vi "Teleop.vi"(10 "Match Info":T2={"Autonomous Elapsed Seconds"=0.0, "TeleOp Elapsed Seconds"=0.0, "Disabled Elapsed Seconds"=0.0, "Visited Autonomous"=FALSE, "Visited TeleOp"=FALSE, "Visited Disabled"=FALSE, "Autonomous Settings"={"Autonomous Style"=enum."Independent", "VI Refnum"=refnum}}, 11 "Call Context":T3) -> ()   [LabVIEW 2012]
doc: "This VI is called for each TeleOp packet received from the DS where the robot is not disabled. It is often used to read from the joysticks and update I/O or to update setpoints for timed control loops. It should complete and return within 20 milliseconds or it may miss DS packets."
uses:
  <vilib>/Rock Robotics/WPI/DriverStation/WPI_DriverStationDerivedRobotMode.ctl
  <vilib>/Rock Robotics/WPI/DriverStation/WPI_DriverStationMatch Info.ctl
  <vilib>/Rock Robotics/WPI/Solenoid/WPI_SolenoidValue.ctl
  Robot Global Data.vi
  <vilib>/addons/control/pid/pid.llb/PID (DBL).vi
  <vilib>/Rock Robotics/WPI/Joystick/WPI_JoystickGetSetRefNum.vi
  <vilib>/Rock Robotics/WPI/RobotDrive/WPI_RobotDriveGetSetRefNum.vi
  <vilib>/Rock Robotics/WPI/Solenoid/WPI_SolenoidSetEnum.vi
  <vilib>/addons/control/pid/NI_PID_pid.lvlib
panel:
  out "Posistioned":string="Nothing"
  out "Angle Target":dbl
  out "Distance From Target":dbl
  out "Ready To Fire":bool
  in  "S Off Time":dbl
  in  "S On Time":dbl
  out "Time Last Fired":dbl
  out "Current Status":string="Roaming"
  in  "Shooter Speed":dbl format="%.2f"
  in  "Shooter On":bool
  out "Waveform Chart":cluster{"Rate":dbl, "Rate":dbl}(graph)
  out "Rate 1":dbl
  out "Rate 2":dbl
  in  "PID gains":T1={"proportional gain (Kc)"=1.0, "integral time (Ti, min)"=0.01, "derivative time (Td, min)"=0.0} {"derivative time (Td, min)" format="%.3f"; "integral time (Ti, min)" format="%.3f"; "proportional gain (Kc)" format="%.3f"}
  in  "Maximum Encoder speed":dbl=25000.0
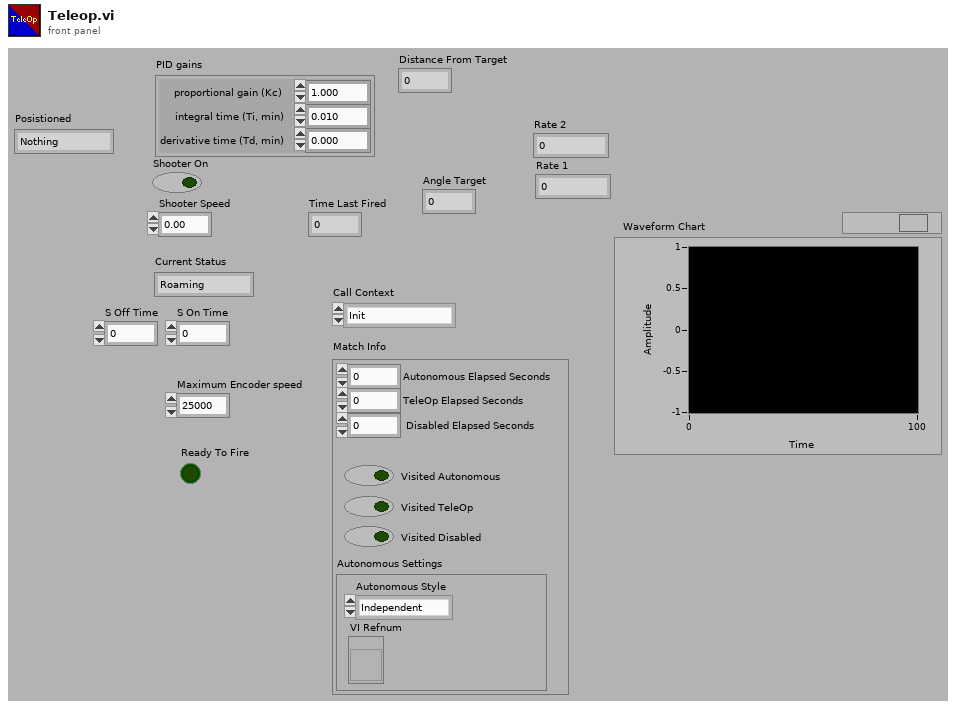
[diagram p1: front panel]
types:
  T1 = cluster{"proportional gain (Kc)":dbl, "integral time (Ti, min)":dbl, "derivative time (Td, min)":dbl}
  T2 = typedef "WPI_DriverStationMatch Info.ctl" = cluster{"Autonomous Elapsed Seconds":dbl, "TeleOp Elapsed Seconds":dbl, "Disabled Elapsed Seconds":dbl, "Visited Autonomous":bool, "Visited TeleOp":bool, "Visited Disabled":bool, "Autonomous Settings":cluster{"Autonomous Style":enum16{"Iterative", "Independent"}, "VI Refnum":refnum<vi>}}
  T3 = typedef "WPI_DriverStationDerivedRobotMode.ctl" = enum16{"Init", "Execute", "Stop"}
  T4 = typedef "WPI_EncoderDevRef.ctl" = cluster{"DevStatus":errorcluster, "EncoderIndex":T5, "CounterIndex":T6, "DistancePerCount":dbl, "Decoding Type":T7}
  T5 = typedef "FPGA_EncoderIdx.ctl" = enum8{"Enc 0", "Enc 1", "Enc 2", "Enc 3", "Invalid"}
  T6 = typedef "FPGA_CounterCtrSystemIndex.ctl" = enum8{"Ctr 0", "Ctr 1", "Ctr 2", "Ctr 3", "Ctr 4", "Ctr 5", "Ctr 6", "Ctr 7", "Invalid"}
  T7 = typedef "WPI_EncoderType.ctl" = enum16{"1x", "2x", "4x"}
  T8 = typedef "WPI_RobotDriveDevRef.ctl" = cluster{"DevStatus":errorcluster, "Motors[]":T9[], "Square Inputs":bool, "Max Output":dbl, "Isochronous":bool}
  T9 = typedef "WPI_MotorControlDeviceRef.ctl" = cluster{"DeviceStatus":errorcluster, "Type":enum16{"PWM", "CAN"}, "PWM":cluster{"Digital Module":T10, "PWM Channel":T11, "DeadBand":T12}, "CAN":cluster{"Device Number":u8, "Control Mode":T13, "Semaphore":T14, "Max Vout":dbl}, "Invert":bool, "TransformRef":T15, "InvTransformRef":T15}
  T10 = typedef "FPGA_TypedefDigitalModule.ctl" = enum16{"Digital Module 1", "Digital Module 2"}
  T11 = typedef "FPGA_DIOPWMChannel.ctl" = enum8{"PWM 1", "PWM 2", "PWM 3", "PWM 4", "PWM 5", "PWM 6", "PWM 7", "PWM 8", "PWM 9", "PWM 10", "Invalid"}
  T12 = typedef "WPI_PWMDeadband.ctl" = cluster{"Name":string, "maxPositivePwm":i32, "minPositivePwm":i32, "centerPwm":i32, "maxNegativePwm":i32, "minNegativePwm":i32, "angularRange":u16}
  T13 = typedef "WPI_CANJaguar_ControlMode.ctl" = enum8{"Percent VBus", "Current", "Speed", "Position", "Voltage"}
  T14 = typedef "Semaphore RefNum" = refnum<k1>
  T15 = typedef "WPI_PWMTransform_ConPane.ctl" = refnum<vi>
  T16 = typedef "WPI_JoystickDevRef.ctl" = cluster{"Device":T17}
  T17 = typedef "WPI_JoystickDeviceEnum.ctl" = enum16{"USB 1", "USB 2", "USB 3", "USB 4", "Kinect 1", "Kinect 2"}
  T18 = typedef "WPI_JoystickButtonState.ctl" = cluster{"Button 1":bool, "Button 2":bool, "Button 3":bool, "Button 4":bool, "Button 5":bool, "Button 6":bool, "Button 7":bool, "Button 8":bool, "Button 9":bool, "Button 10":bool, "Button 11":bool, "Button 12":bool}
  T19 = cluster{"axis 1 (x)":dbl, "axis 2 (y)":dbl, "axis 3 (throttle)":dbl, "axis 4":dbl, "axis 5":dbl, "axis 6":dbl}
  T20 = typedef "WPI_SolenoidValue.ctl" = enum16{"Off", "On", "Forward", "Reverse"}
  T21 = typedef "WPI_SolenoidDevRef.ctl" = cluster{"DevStatus":errorcluster, "Solenoid Module":T22, "Forward Solenoid Channel":T23, "Reverse Solenoid Channel":T23}
  T22 = typedef "FPGA_TypedefSolenoidModule.ctl" = enum16{"Solenoid Module 1", "Solenoid Module 2"}
  T23 = typedef "WPI_SolenoidChannel.ctl" = enum8{"Solenoid 1", "Solenoid 2", "Solenoid 3", "Solenoid 4", "Solenoid 5", "Solenoid 6", "Solenoid 7", "Solenoid 8", "Invalid"}
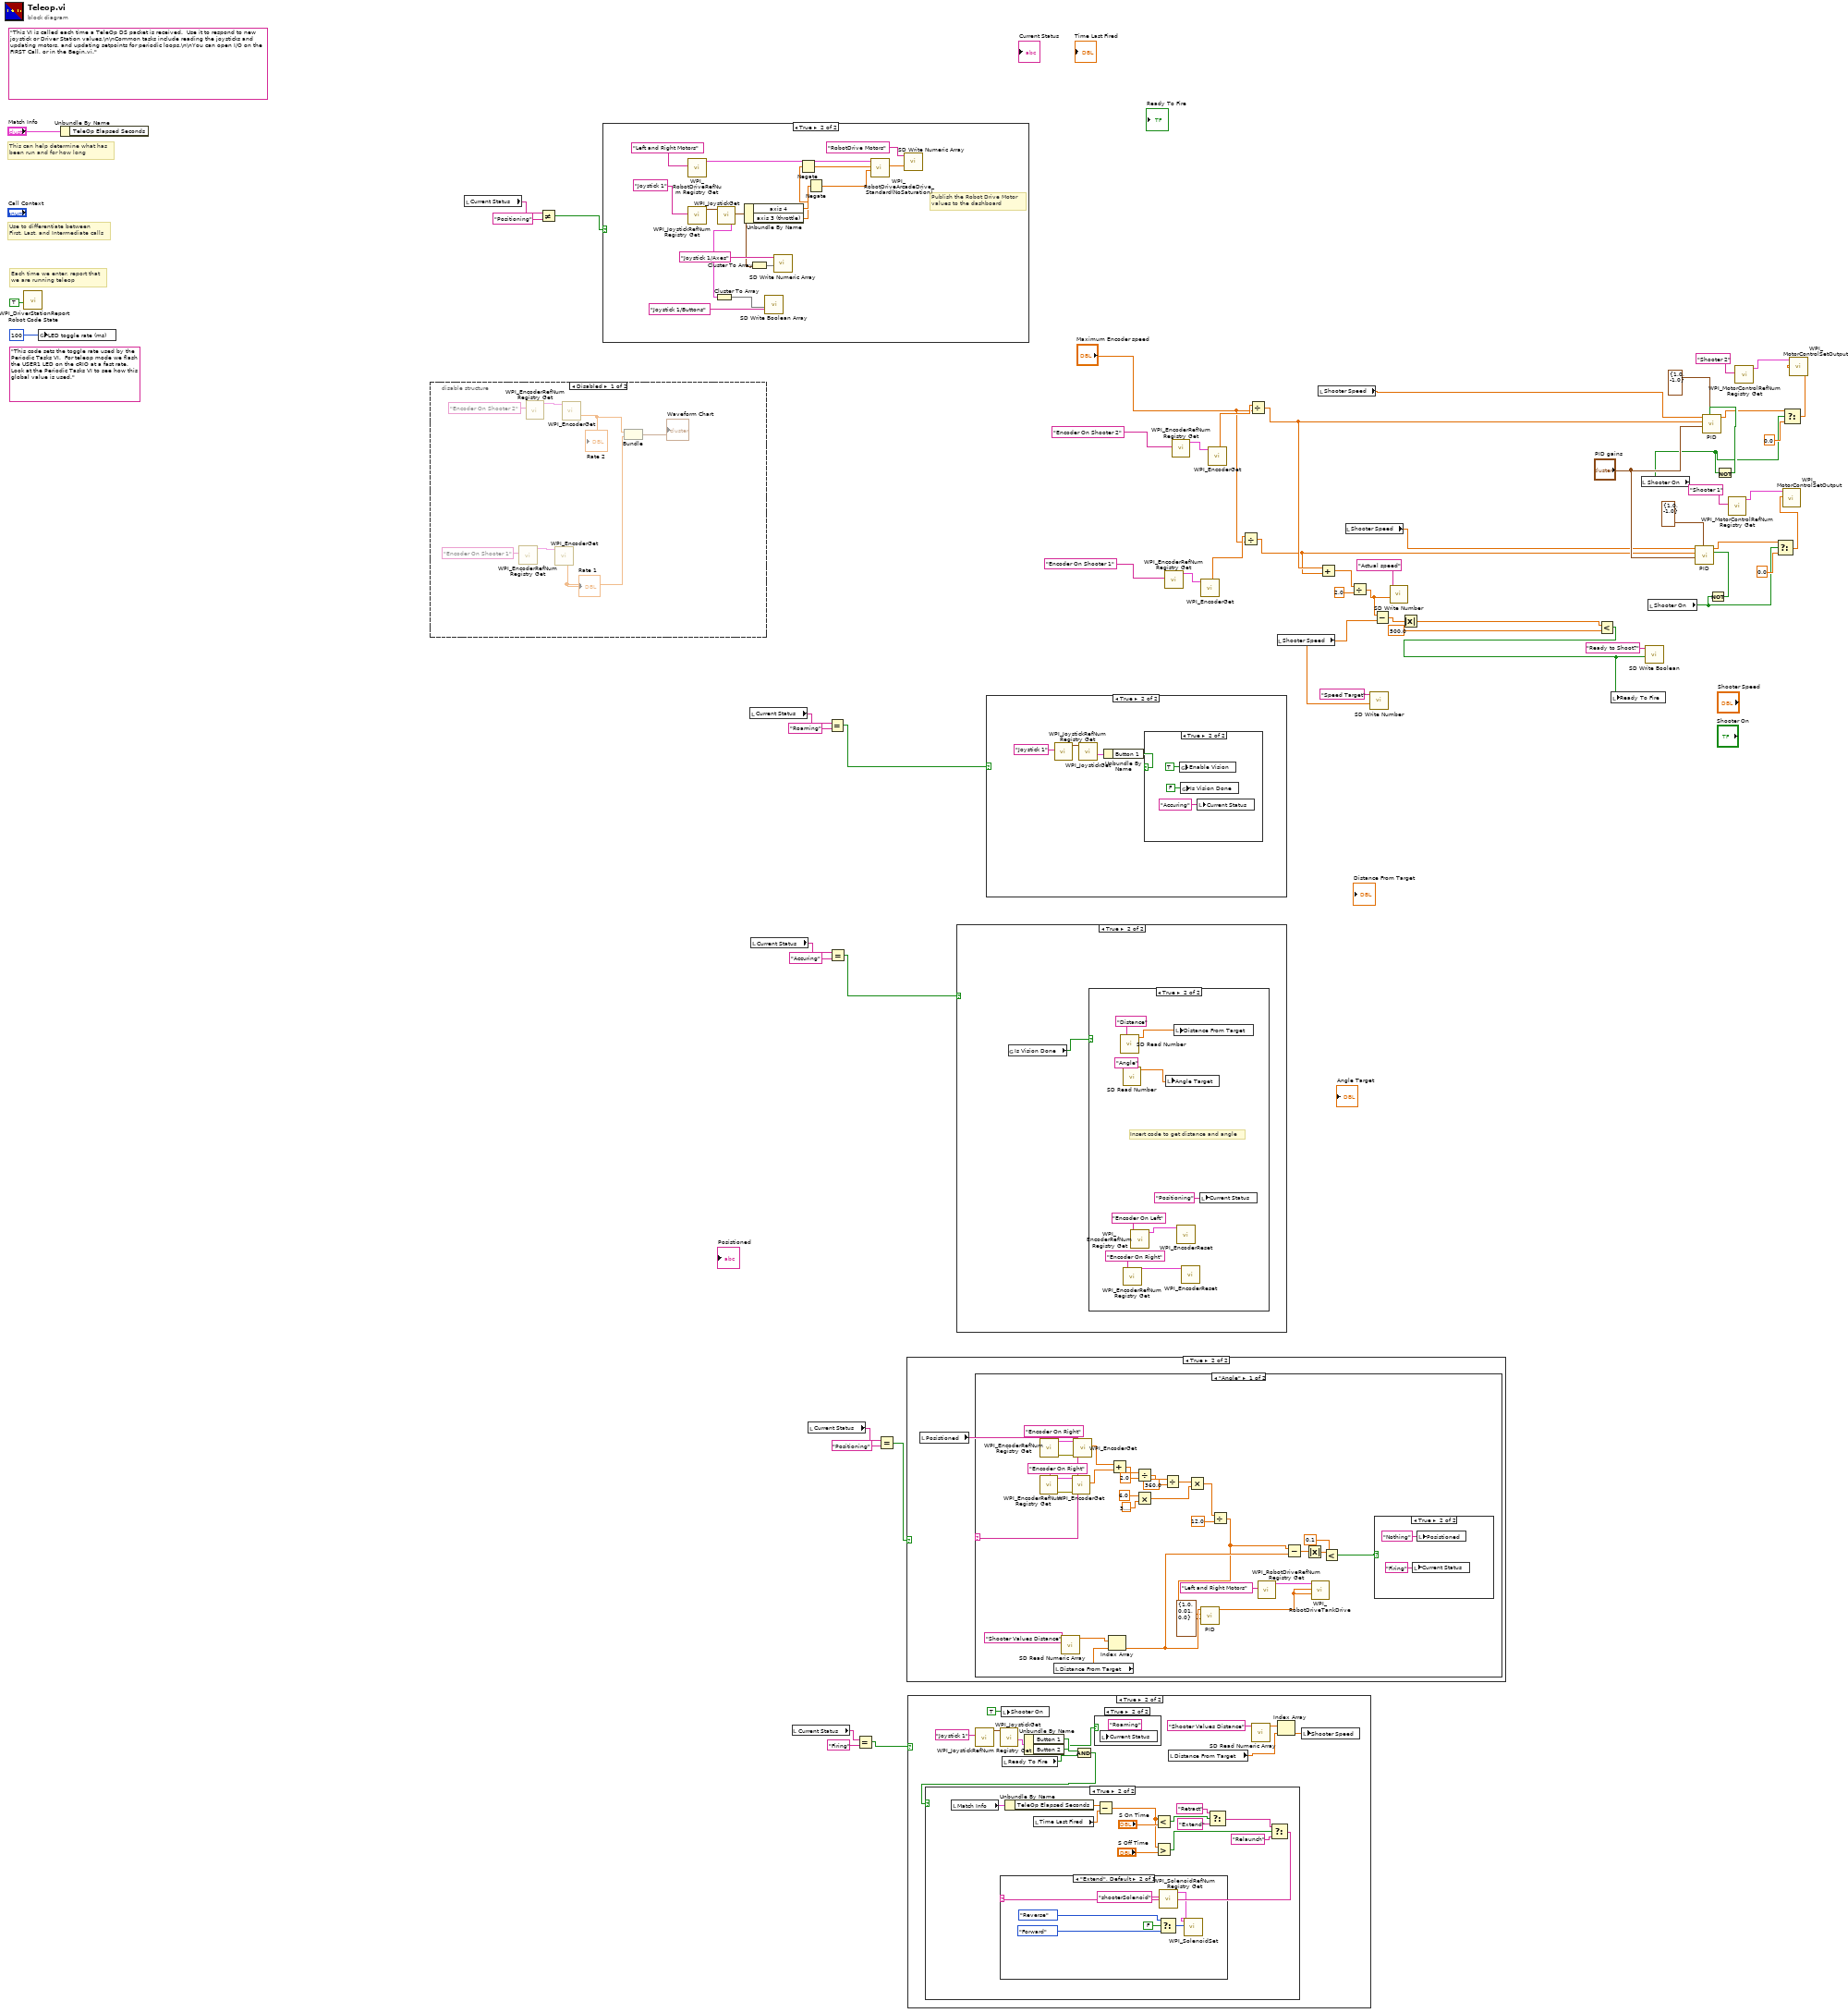
[diagram p0: block diagram]
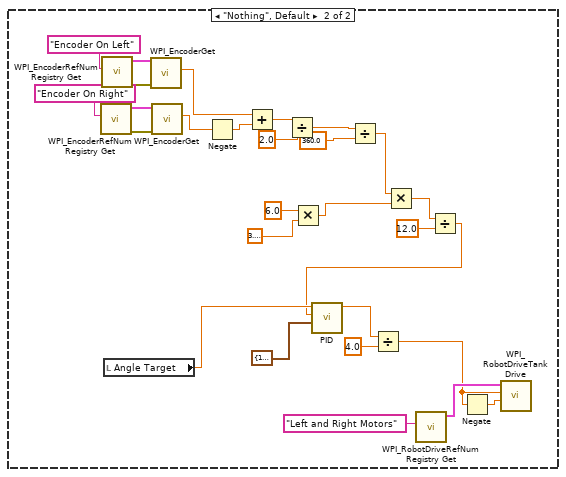
[diagram p4: hidden frame]
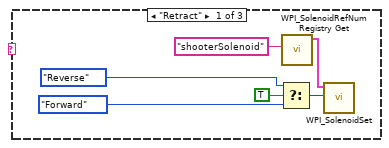
[diagram p13: hidden frame]
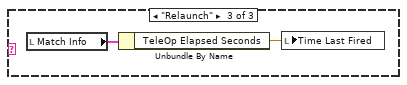
[diagram p14: hidden frame]
diagram:
  (unwired) "This code sets the toggle rate used by the Periodic Tasks VI.  For teleop mode we flash the USER1 LED on the cRIO at a fast rate.  Look at the Periodic Tasks VI to see how this global value is used."
  (unwired) "This VI is called each time a TeleOp DS packet is received.  Use it to respond to new joystick or Driver Station values.\n\nCommon tasks include reading the joysticks and updating motors, and updating setpoints for periodic loops.\n\nYou can open I/O on the FIRST Call, or in the Begin.vi."
  # "Each time we enter, report that\nwe are running teleop"
  # "Use to differentiate between\nFirst, Last, and Intermediate calls"
  # "This can help determine what has\nbeen run and for how long"
  n1 = call <vilib>:"WPI_DriverStationReport Robot Code State.vi"("TeleOp"=TRUE ("Autonomous")) -> ()  [unwired: 10 in, 1 out]
  n2 = global write "Robot Global Data.vi" "LED toggle rate (ms)"(u32 100 ("LED ms toggle rate")) -> ()
  n3 = Unbundle By Name("Match Info") -> ()  [unwired: 1 out]
  n4 = disable-structure shown="Disabled" {
    frame Disabled {
      n5 = call <vilib>:"WPI_EncoderRefNum Registry Get.vi"("refnum name"="Encoder On Shooter 1") -> ("EncoderDevRef"=w62:T4)  [unwired: 9 in, 1 out]
      n6 = call <vilib>:"WPI_EncoderRefNum Registry Get.vi"("refnum name"="Encoder On Shooter 2") -> ("EncoderDevRef"=w63:T4)  [unwired: 9 in, 1 out]
      n7 = call <vilib>:"WPI_EncoderGet.vi"("EncoderDevRef"=w62) -> ("Rate"=w61:dbl)  [unwired: 5 in, 5 out]
      "Rate 1" <- w61
      n8 = call <vilib>:"WPI_EncoderGet.vi"("EncoderDevRef"=w63) -> ("Rate"=w60:dbl)  [unwired: 5 in, 5 out]
      "Rate 2" <- w60
      n9 = Bundle("Rate"=w60, "Rate"=w61) -> (→"Waveform Chart":cluster{"Rate":dbl, "Rate":dbl})  [unwired: 1 in]
    }
    frame Enabled {
    }
  }
  n10 = local read "Current Status"() -> (w6:string)
  n11 = Not Equal?(x=w6, y="Positioning") -> (x != y?=w4:bool)
  n12 = case shown="True" w4 {
    frame False {
    }
    frame True {
      # "Publish the Robot Drive Motor\nvalues to the dashboard"
      n13 = call <vilib>:"WPI_RobotDriveRefNum Registry Get.vi"("refnum name"="Left and Right Motors") -> ("RobotDriveDevRef"=w71:T8)  [unwired: 1 in, 9 out]
      n14 = call <vilib>:"WPI_JoystickRefNum Registry Get.vi"("refnum name"="Joystick 1") -> ("JoystickDevRef"=w72:T16)  [unwired: 1 in, 9 out]
      n15 = call <vilib>:"WPI_JoystickGet.vi"("JoystickDevRef"=w72) -> ("Buttons"=w73:T18, "Axes"=w76:T19)  [unwired: 1 in, 4 out]
      n16 = Cluster To Array(cluster=w73) -> (array=w74:bool[])
      n17 = Unbundle By Name(w76) -> ("axis 4"=w68:dbl, "axis 3 (throttle)"=w65:dbl)
      n18 = Cluster To Array(cluster=w76) -> (array=w77:dbl[])
      n19 = call <vilib>:"SD Write Boolean Array.vi"("Boolean Array"=w74, "Name"="Joystick 1/Buttons") -> ()  [unwired: 8 in, 2 out]
      n20 = call <vilib>:"SD Write Numeric Array.vi"("Numeric Array"=w77, "Name"="Joystick 1/Axes") -> ()  [unwired: 8 in, 2 out]
      n21 = Negate(x=w68) -> (-x=w67:dbl)
      n22 = Negate(x=w65) -> (-x=w66:dbl)
      n23 = call <vilib>:"WPI_RobotDriveArcadeDrive_Standard(NoSaturation).vi"("Y axis value"=w66, "X axis value"=w67, "RobotDriveDevRef"=w71) -> ("Motor Values"=w80:dbl[])  [unwired: 1 in, 7 out]
      n24 = call <vilib>:"SD Write Numeric Array.vi"("Numeric Array"=w80, "Name"="RobotDrive Motors") -> ()  [unwired: 8 in, 2 out]
    }
  }
  n25 = local read "Current Status"() -> (w12:string)
  n26 = local read "Current Status"() -> (w9:string)
  n27 = local read "Current Status"() -> (w28:string)
  n28 = local read "Current Status"() -> (w3:string)
  n29 = Equal?(x=w12, y="Roaming") -> (x = y?=w10:bool)
  n30 = Equal?(x=w9, y="Accuring") -> (x = y?=w7:bool)
  n31 = Equal?(x=w28, y="Firing") -> (x = y?=w26:bool)
  n32 = Equal?(x=w3, y="Positioning") -> (x = y?=w1:bool)
  n33 = case shown="True" w1 {
    frame False {
    }
    frame True {
      n34 = local read "Posistioned"() -> (w81:string)
      n35 = case shown="\"Angle\"" w81 {
        frame "Angle" {
          n36 = call <vilib>:"WPI_EncoderRefNum Registry Get.vi"("refnum name"="Encoder On Right") -> ("error out"=w84:errorcluster, "EncoderDevRef"=w85:T4)  [unwired: 9 in]
          n37 = call <vilib>:"WPI_EncoderRefNum Registry Get.vi"("refnum name"="Encoder On Right") -> ("error out"=w82:errorcluster, "EncoderDevRef"=w83:T4)  [unwired: 9 in]
          n38 = local read "Distance From Target"() -> (w105:dbl)
          n39 = call <vilib>:"SD Read Numeric Array.vi"("Name"="Shooter Values Distance") -> ("Numeric Array"=w104:dbl[])  [unwired: 8 in, 2 out]
          n40 = call <vilib>:"WPI_EncoderGet.vi"("error in (no error)"=w84, "EncoderDevRef"=w85) -> ("Distance"=w89:dbl)  [unwired: 4 in, 5 out]
          n41 = call <vilib>:"WPI_EncoderGet.vi"("error in (no error)"=w82, "EncoderDevRef"=w83) -> ("Distance"=w88:dbl)  [unwired: 4 in, 5 out]
          n42 = Index Array(array=w104, index=w105) -> (element=w109:dbl)
          n43 = Add(x=w88, y=w89) -> (x+y=w90:dbl)
          n44 = Divide(x=w90, y=2.0) -> (x/y=w94:dbl)
          n45 = Multiply(x=6.0, y=3.141592653589793) -> (x*y=w97:dbl)
          n46 = Divide(x=w94, y=360.0) -> (x/y=w96:dbl)
          n47 = Multiply(x=w96, y=w97) -> (x*y=w98:dbl)
          n48 = Divide(x=w98, y=12.0) -> (x/y=w108:dbl)
          n49 = call-poly <vilib>:"PID.vi"("PID gains"=T1 {"proportional gain (Kc)"=1.0, "integral time (Ti, min)"=0.01, "derivative time (Td, min)"=0.0}, "process variable"=w108, "setpoint"=w109) -> ("output"=w102:dbl)  [unwired: 7 in, 1 out]
          n50 = call <vilib>:"WPI_RobotDriveRefNum Registry Get.vi"("refnum name"="Left and Right Motors") -> ("RobotDriveDevRef"=w101:T8)  [unwired: 9 in, 1 out]
          n51 = Subtract(x=w108, y=w109) -> (x-y=w107:dbl)
          n52 = Absolute Value(x=w107) -> (abs(x)=w110:dbl)
          n53 = call <vilib>:"WPI_RobotDriveTankDrive.vi"("Right axis value"=w102, "Left axis value"=w102, "RobotDriveDevRef"=w101) -> ()  [unwired: 6 in, 3 out]
          n54 = Less?(x=w110, y=0.1) -> (x < y?=w112:bool)
          n55 = case shown="True" w112 {
            frame False {
            }
            frame True {
              n56 = local write "Current Status"("Firing" ("Current Status")) -> ()
              n57 = local write "Posistioned"("Nothing" ("Posistioned")) -> ()
            }
          }
        }
        frame "Nothing", Default {
          n58 = call <vilib>:"WPI_EncoderRefNum Registry Get.vi"("refnum name"="Encoder On Right") -> ("error out"=w140:errorcluster, "EncoderDevRef"=w139:T4)  [unwired: 9 in]
          n59 = call <vilib>:"WPI_EncoderRefNum Registry Get.vi"("refnum name"="Encoder On Left") -> ("error out"=w142:errorcluster, "EncoderDevRef"=w141:T4)  [unwired: 9 in]
          n60 = local read "Angle Target"() -> (w131:dbl)
          n61 = call <vilib>:"WPI_EncoderGet.vi"("error in (no error)"=w142, "EncoderDevRef"=w141) -> ("Distance"=w135:dbl)  [unwired: 4 in, 5 out]
          n62 = call <vilib>:"WPI_EncoderGet.vi"("error in (no error)"=w140, "EncoderDevRef"=w139) -> ("Distance"=w136:dbl)  [unwired: 4 in, 5 out]
          n63 = Negate(x=w136) -> (-x=w134:dbl)
          n64 = Add(x=w135, y=w134) -> (x+y=w133:dbl)
          n65 = Divide(x=w133, y=2.0) -> (x/y=w128:dbl)
          n66 = Multiply(x=6.0, y=3.141592653589793) -> (x*y=w126:dbl)
          n67 = Divide(x=w128, y=360.0) -> (x/y=w115:dbl)
          n68 = Multiply(x=w115, y=w126) -> (x*y=w125:dbl)
          n69 = call <vilib>:"WPI_RobotDriveRefNum Registry Get.vi"("refnum name"="Left and Right Motors") -> ("RobotDriveDevRef"=w120:T8)  [unwired: 9 in, 1 out]
          n70 = Divide(x=w125, y=12.0) -> (x/y=w123:dbl)
          n71 = call-poly <vilib>:"PID.vi"("PID gains"=T1 {"proportional gain (Kc)"=1.0, "integral time (Ti, min)"=0.01, "derivative time (Td, min)"=0.0}, "process variable"=w123, "setpoint"=w131) -> ("output"=w117:dbl)  [unwired: 7 in, 1 out]
          n72 = Divide(x=w117, y=4.0) -> (x/y=w116:dbl)
          n73 = Negate(x=w116) -> (-x=w119:dbl)
          n74 = call <vilib>:"WPI_RobotDriveTankDrive.vi"("Right axis value"=w119, "Left axis value"=w116, "RobotDriveDevRef"=w120) -> ()  [unwired: 6 in, 3 out]
        }
      }
    }
  }
  n75 = case shown="True" w26 {
    frame False {
    }
    frame True {
      n76 = call <vilib>:"WPI_JoystickRefNum Registry Get.vi"("refnum name"="Joystick 1") -> ("JoystickDevRef"=w150:T16)  [unwired: 9 in, 1 out]
      n77 = call <vilib>:"WPI_JoystickGet.vi"("JoystickDevRef"=w150) -> ("Buttons"=w149:T18)  [unwired: 4 in, 2 out]
      n78 = local write "Shooter On"(TRUE ("Shooter On")) -> ()
      n79 = local read "Ready To Fire"() -> (w146:bool)
      n80 = Unbundle By Name(w149) -> ("Button 1"=w148:bool, "Button 2"=w143:bool)
      n81 = And(x=w148, y=w146) -> (x .and. y?=w147:bool)
      n82 = case shown="True" w147 {
        frame False {
        }
        frame True {
          n83 = local read "Match Info"() -> (w168:T2)
          n84 = Unbundle By Name(w168) -> ("TeleOp Elapsed Seconds"=w167:dbl)
          n85 = local read "Time Last Fired"() -> (w166:dbl)
          n86 = Subtract(x=w167, y=w166) -> (x-y=w158:dbl)
          n87 = Less?(x=w158, y="S On Time") -> (x < y?=w162:bool)
          n88 = Greater?(x=w158, y="S Off Time") -> (0:w156:bool)
          n89 = Select(t="Retract" ("f"), s=w162, f="Extend") -> (s? t:f=w159:string)
          n90 = Select(t=w159, s=w156, f="Relaunch") -> (s? t:f=w163:string)
          n91 = case shown="\"Extend\", Default" w163 {
            frame "Retract" {
              n92 = Select(t=WPI_SolenoidValue."Reverse" ("Value"), s=TRUE, f=WPI_SolenoidValue."Forward" ("Value")) -> (s? t:f=w173:T20)
              n93 = call <vilib>:"WPI_SolenoidRefNum Registry Get.vi"("refnum name"="shooterSolenoid") -> ("SolenoidDevRef"=w169:T21)  [unwired: 9 in, 1 out]
              n94 = call-poly <vilib>:"WPI_SolenoidSet.vi"("Value"=w173, "SolenoidDevRef"=w169) -> ()  [unwired: 8 in, 2 out]
            }
            frame "Extend", Default {
              n95 = Select(t=WPI_SolenoidValue."Reverse" ("Value"), s=FALSE, f=WPI_SolenoidValue."Forward" ("Value")) -> (s? t:f=w179:T20)
              n96 = call <vilib>:"WPI_SolenoidRefNum Registry Get.vi"("refnum name"="shooterSolenoid") -> ("SolenoidDevRef"=w175:T21)  [unwired: 9 in, 1 out]
              n97 = call-poly <vilib>:"WPI_SolenoidSet.vi"("Value"=w179, "SolenoidDevRef"=w175) -> ()  [unwired: 8 in, 2 out]
            }
            frame "Relaunch" {
              n98 = local read "Match Info"() -> (w182:T2)
              n99 = Unbundle By Name(w182) -> ("TeleOp Elapsed Seconds"=w181:dbl)
              n100 = local write "Time Last Fired"(w181) -> ()
            }
          }
        }
      }
      n101 = case shown="True" w143 {
        frame False {
        }
        frame True {
          n102 = local write "Current Status"("Roaming" ("Current Status")) -> ()
        }
      }
      n103 = local read "Distance From Target"() -> (w144:dbl)
      n104 = call <vilib>:"SD Read Numeric Array.vi"("Name"="Shooter Values Distance") -> ("Numeric Array"=w153:dbl[])  [unwired: 8 in, 2 out]
      n105 = Index Array(array=w153, index=w144) -> (element=w152:dbl)
      n106 = local write "Shooter Speed"(w152) -> ()
    }
  }
  n107 = case shown="True" w7 {
    frame False {
    }
    frame True {
      n108 = global read "Robot Global Data.vi" "Is Vision Done"() -> (w183:bool)
      n109 = case shown="True" w183 {
        frame False {
        }
        frame True {
          # "Insert code to get distance and angle"
          n110 = call <vilib>:"SD Read Number.vi"("Name"="Distance") -> ("Numeric"=w190:dbl)  [unwired: 8 in, 2 out]
          n111 = call <vilib>:"SD Read Number.vi"("Name"="Angle") -> ("Numeric"=w184:dbl)  [unwired: 8 in, 2 out]
          n112 = call <vilib>:"WPI_EncoderRefNum Registry Get.vi"("refnum name"="Encoder On Right") -> ("EncoderDevRef"=w187:T4)  [unwired: 9 in, 1 out]
          n113 = call <vilib>:"WPI_EncoderRefNum Registry Get.vi"("refnum name"="Encoder On Left") -> ("EncoderDevRef"=w188:T4)  [unwired: 9 in, 1 out]
          n114 = local write "Angle Target"(w184) -> ()
          n115 = local write "Distance From Target"(w190) -> ()
          n116 = call <vilib>:"WPI_EncoderReset.vi"("EncoderDevRef"=w188) -> ()  [unwired: 9 in, 2 out]
          n117 = call <vilib>:"WPI_EncoderReset.vi"("EncoderDevRef"=w187) -> ()  [unwired: 9 in, 2 out]
          n118 = local write "Current Status"("Positioning" ("Current Status")) -> ()
        }
      }
    }
  }
  n119 = case shown="True" w10 {
    frame False {
    }
    frame True {
      n120 = call <vilib>:"WPI_JoystickRefNum Registry Get.vi"("refnum name"="Joystick 1") -> ("JoystickDevRef"=w195:T16)  [unwired: 9 in, 1 out]
      n121 = call <vilib>:"WPI_JoystickGet.vi"("JoystickDevRef"=w195) -> ("Buttons"=w194:T18)  [unwired: 4 in, 2 out]
      n122 = Unbundle By Name(w194) -> ("Button 1"=w193:bool)
      n123 = case shown="True" w193 {
        frame False {
        }
        frame True {
          n124 = global write "Robot Global Data.vi" "Enable Vision"(TRUE ("Enable Vision")) -> ()
          n125 = global write "Robot Global Data.vi" "Is Vision Done"(FALSE ("Is Vision Done")) -> ()
          n126 = local write "Current Status"("Accuring" ("Current Status")) -> ()
        }
      }
    }
  }
  n127 = call <vilib>:"WPI_EncoderRefNum Registry Get.vi"("refnum name"="Encoder On Shooter 1") -> ("EncoderDevRef"=w51:T4)  [unwired: 9 in, 1 out]
  n128 = call <vilib>:"WPI_EncoderRefNum Registry Get.vi"("refnum name"="Encoder On Shooter 2") -> ("EncoderDevRef"=w42:T4)  [unwired: 9 in, 1 out]
  n129 = call <vilib>:"WPI_EncoderGet.vi"("EncoderDevRef"=w51) -> ("Rate"=w35:dbl)  [unwired: 5 in, 5 out]
  n130 = call <vilib>:"WPI_EncoderGet.vi"("EncoderDevRef"=w42) -> ("Rate"=w34:dbl)  [unwired: 5 in, 5 out]
  n131 = Divide(x=w35, y="Maximum Encoder speed") -> (x/y=w23:dbl)
  n132 = Divide(x=w34, y="Maximum Encoder speed") -> (x/y=w24:dbl)
  n133 = local read "Shooter Speed"() -> (w19:dbl)
  n134 = local read "Shooter Speed"() -> (w29:dbl)
  n135 = Add(x=w24, y=w23) -> (x+y=w22:dbl)
  n136 = local read "Shooter Speed"() -> (w30:dbl)
  n137 = Divide(x=w22, y=2.0) -> (x/y=w18:dbl)
  n138 = call <vilib>:"SD Write Number.vi"("Numeric"=w19, "Name"="Speed Target") -> ()  [unwired: 8 in, 2 out]
  n139 = Subtract(x=w18, y=w19) -> (x-y=w17:dbl)
  n140 = call <vilib>:"SD Write Number.vi"("Numeric"=w18, "Name"="Actual speed") -> ()  [unwired: 8 in, 2 out]
  n141 = Absolute Value(x=w17) -> (abs(x)=w16:dbl)
  n142 = Less?(x=w16, y=500.0) -> (x < y?=w13:bool)
  n143 = local write "Ready To Fire"(w13) -> ()
  n144 = local read "Shooter On"() -> (w32:bool)
  n145 = call <vilib>:"SD Write Boolean.vi"("Boolean"=w13, "Name"="Ready to Shoot?") -> ()  [unwired: 8 in, 2 out]
  n146 = local read "Shooter On"() -> (w31:bool)
  n147 = Not(x=w31) -> (.not. x?=w53:bool)
  n148 = call-poly <vilib>:"PID.vi"("reinitialize? (F)"=w53, "output range"=cluster{"output high":dbl, "output low":dbl} {"output high"=1.0, "output low"=-1.0}, "PID gains"="PID gains", "process variable"=w23, "setpoint"=w30) -> ("output"=w52:dbl)  [unwired: 5 in, 1 out]
  n149 = Not(x=w32) -> (.not. x?=w44:bool)
  n150 = call-poly <vilib>:"PID.vi"("reinitialize? (F)"=w44, "output range"=cluster{"output high":dbl, "output low":dbl} {"output high"=1.0, "output low"=-1.0}, "PID gains"="PID gains", "process variable"=w24, "setpoint"=w29) -> ("output"=w43:dbl)  [unwired: 5 in, 1 out]
  n151 = call <vilib>:"WPI_MotorControlRefNum Registry Get.vi"("refnum name"="Shooter 1") -> ("MotorControlDevRef"=w46:T9)  [unwired: 9 in, 1 out]
  n152 = call <vilib>:"WPI_MotorControlRefNum Registry Get.vi"("refnum name"="Shooter 2") -> ("MotorControlDevRef"=w37:T9)  [unwired: 9 in, 1 out]
  n153 = Select(t=w52, s=w31, f=0.0) -> (s? t:f=w48:dbl)
  n154 = call <vilib>:"WPI_MotorControlSetOutput.vi"("Output"=w48, "MotorControlDevRef"=w46) -> ()  [unwired: 7 in, 3 out]
  n155 = Select(t=w43, s=w32, f=0.0) -> (s? t:f=w39:dbl)
  n156 = call <vilib>:"WPI_MotorControlSetOutput.vi"("Output"=w39, "MotorControlDevRef"=w37) -> ()  [unwired: 7 in, 3 out]
